vi "Cross Baseline.vi"(8 "error in (no error)":errorcluster, 9 "Scale Factor":sgl, 10 "Speed (ft/s)":dbl, 11 "Team Blue?":bool) -> (0 "error out":errorcluster)   [LabVIEW 2016]
uses:
  <vilib>/Rock Robotics/WPI/RobotDrive/WPI_RobotDriveMecanumDrive_Cartesian.vi
  Global 4.vi
  <vilib>/vision/NI_Vision_Development_Module.lvlib
panel:
  out "X Limit":i32
  out "Y Limit":i32
  out "BrightestY":i32
  out "BrightestX":i32
  out "Brightestness":u16
  in  "Control Brightness":u16
  in  "Target Brightness":u16
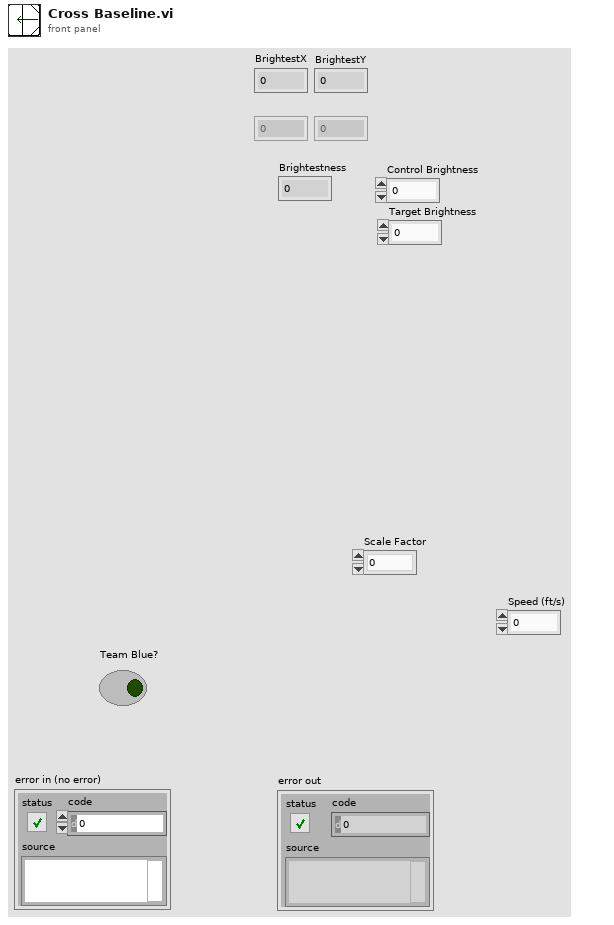
[diagram p1: front panel]
types:
  T1 = typedef "IMAQ Image.ctl" = refnum<image>
  T2 = typedef "WPI_RobotDriveDevRef.ctl" = cluster{"DevStatus":errorcluster, "Motors[]":T3[], "Square Inputs":bool, "Max Output":dbl}
  T3 = typedef "WPI_MotorControlDeviceRef.ctl" = cluster{"DeviceStatus":errorcluster, "Type":T4, "PWM":cluster{"PWM Channel":T5, "DeadBand":T6}, "CAN":cluster{"Device Number":u8, "SetOutput VI Ref":variant, "GetOutput VI Ref":variant, "Enable VI Ref":variant, "Disable VI Ref":variant, "Data":variant}, "Invert":bool}
  T4 = typedef "WPI_MotorControlType.ctl" = enum16{"PWM", "CAN"}
  T5 = typedef "FPGA_DIOPWMChannel.ctl" = enum8{"PWM 0", "PWM 1", "PWM 2", "PWM 3", "PWM 4", "PWM 5", "PWM 6", "PWM 7", "PWM 8", "PWM 9", "PWM MXP 0", "PWM MXP 1", "PWM MXP 2", "PWM MXP 3", "PWM MXP 4", "PWM MXP 5", "PWM MXP 6", "PWM MXP 7", "PWM MXP 8", "PWM MXP 9", "Invalid"}
  T6 = typedef "WPI_PWMDeadband.ctl" = cluster{"Name":string, "maxPositivePwm":i32, "minPositivePwm":i32, "centerPwm":i32, "maxNegativePwm":i32, "minNegativePwm":i32, "angularRange":u16}
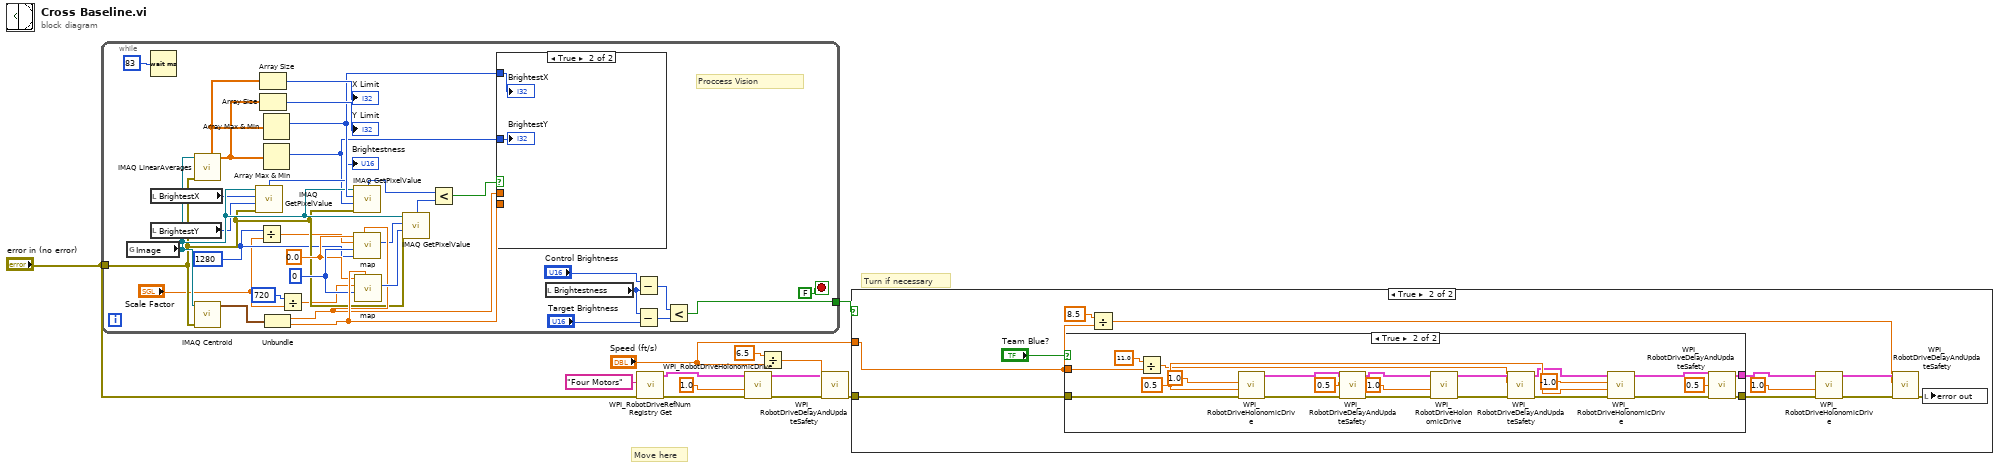
[diagram p0: block diagram]
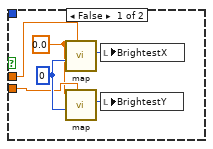
[diagram p2: hidden frame]
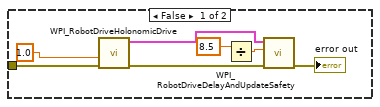
[diagram p3: hidden frame]
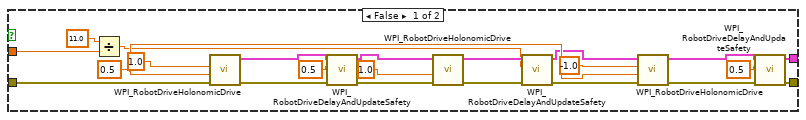
[diagram p4: hidden frame]
diagram:
  # "Turn if necessary"
  # "Move here"
  n1 = while {
    tunnel: "error in (no error)" -> [w19]
    tunnel: [w13] -> w12
    stop <- FALSE stop-if-true
    w17 = 1280
    w20 = sgl 0.0
    w21 = 0
    # "Proccess Vision"
    n2 = global read "Global 4.vi" "Image"() -> (w39:T1)
    n3 = Wait (ms)(milliseconds to wait=u32 83) -> ()  [unwired: 1 out]
    n4 = local read "BrightestX"() -> (w38:i32)
    n5 = local read "BrightestY"() -> (w37:i32)
    n6 = call "IMAQ LinearAverages"("error in (no error)"=w19, "Image Src"=w39) -> ("Y Axis Averages"=w42:sgl[], "X Axis Averages"=w43:sgl[])  [unwired: 5 in, 3 out]
    n7 = call "IMAQ Centroid"("error in (no error)"=w19, "Image"=w39) -> ("Centroid"=w44:cluster{"X Centroid":sgl, "Y Centroid":sgl})  [unwired: 2 in, 1 out]
    n8 = call "IMAQ GetPixelValue"("Image"=w39, "X Coordinate"=w38, "Y Coordinate"=w37, "error in (no error)"=w19) -> ("Pixel Value (U16)"=→"Brightestness":u16)  [unwired: 2 in, 4 out]
    n9 = Divide(x=w17, y="Scale Factor") -> (x/y=w18:sgl)
    n10 = Array Size(array=w43) -> (size(s)=→"X Limit":i32)
    n11 = Array Size(array=w42) -> (size(s)=→"Y Limit":i32)
    n12 = Array Max & Min(array=w43) -> (max index (indices)=w40:i32)  [unwired: 3 out]
    n13 = Array Max & Min(array=w42) -> (max index (indices)=w28:i32)  [unwired: 3 out]
    n14 = Unbundle(w44) -> ("X Centroid"=w23:sgl, "Y Centroid"=w25:sgl)
    n15 = Divide(x=720, y="Scale Factor") -> (x/y=w14:sgl)
    n16 = call "IMAQ GetPixelValue"("Image"=w39, "X Coordinate"=w40, "Y Coordinate"=w28, "error in (no error)"=w19) -> ("Pixel Value (U16)"=w33:u16)  [unwired: 2 in, 4 out]
    n17 = call "map.vi"("value"=w23, "newMax"=w17, "newMin"=w21, "oldMax"=w18, "oldMin"=w20) -> ("newValue"=w22:i32)  [unwired: 6 in]
    n18 = call "map.vi"("value"=w25, "newMin"=w21, "oldMax"=w14, "oldMin"=w20) -> ("newValue"=w24:i32)  [unwired: 7 in]
    n19 = call "IMAQ GetPixelValue"("Image"=w39, "X Coordinate"=w22, "Y Coordinate"=w24, "error in (no error)"=w19) -> ("Pixel Value (U16)"=w32:u16)  [unwired: 2 in, 4 out]
    n20 = Less?(x=w33, y=w32) -> (x < y?=w41:bool)
    n21 = case shown="True" w41 {
      tunnel: w40 -> [_ w54]
      tunnel: w23 -> [w52 _]
      tunnel: w25 -> [w49 _]
      tunnel: w28 -> [_ w53]
      frame False {
        w50 = 0
        w48 = sgl 0.0
        n22 = call "map.vi"("value"=w52, "newMin"=w50, "oldMin"=w48) -> ("newValue"=w51:i32)  [unwired: 8 in]
        n23 = call "map.vi"("value"=w49, "newMin"=w50, "oldMin"=w48) -> ("newValue"=w47:i32)  [unwired: 8 in]
        n24 = local write "BrightestX"(w51) -> ()
        n25 = local write "BrightestY"(w47) -> ()
      }
      frame True {
        "BrightestY" <- w53
        "BrightestX" <- w54
      }
    }
    n26 = local read "Brightestness"() -> (w36:u16)
    n27 = Subtract(x="Control Brightness", y=w36) -> (x-y=w29:u16)
    n28 = Subtract(x=w36, y="Target Brightness") -> (x-y=w30:u16)
    n29 = Less?(x=w29, y=w30) -> (x < y?=w13:bool)
  }
  n30 = call <vilib>:"WPI_RobotDriveRefNum Registry Get.vi"("error in (no error)"="error in (no error)", "refnum name"="Four Motors") -> ("error out"=w4:errorcluster, "RobotDriveDevRef"=w5:T2)  [unwired: 8 in]
  n31 = call-poly <vilib>:"WPI_RobotDriveHolonomicDrive.vi"("error in (no error)"=w4, "Y"=1.0, "RobotDriveDevRef"=w5) -> ("error out"=w9:errorcluster, "RobotDriveDevRef"=w8:T2)  [unwired: 6 in, 1 out]
  n32 = Divide(x=6.5, y="Speed (ft/s)") -> (x/y=w10:dbl)
  n33 = call <vilib>:"WPI_RobotDriveDelayAndUpdateSafety.vi"("error in (no error)"=w9, "Delay (s)"=w10, "RobotDriveDevRef"=w8) -> ("error out"=w2:errorcluster)  [unwired: 7 in, 1 out]
  n34 = case shown="True" w12 {
    tunnel: w2 -> [w57 w63]
    tunnel: "Speed (ft/s)" -> [_ w62]
    frame False {
      n35 = call-poly <vilib>:"WPI_RobotDriveHolonomicDrive.vi"("error in (no error)"=w57, "Y"=1.0) -> ("error out"=w60:errorcluster, "RobotDriveDevRef"=w59:T2)  [unwired: 7 in, 1 out]
      n36 = Divide(x=8.5) -> (x/y=w56:dbl)  [unwired: 1 in]
      n37 = call <vilib>:"WPI_RobotDriveDelayAndUpdateSafety.vi"("error in (no error)"=w60, "Delay (s)"=w56, "RobotDriveDevRef"=w59) -> ("error out"=→"error out":errorcluster)  [unwired: 7 in, 1 out]
    }
    frame True {
      n38 = case shown="True" "Team Blue?" {
        tunnel: [w79 w100] -> w72
        tunnel: [w78 w99] -> w71
        tunnel: w63 -> [w75 w97]
        tunnel: w62 -> [w73 w95]
        frame False {
          w84 = 0.5
          n39 = Divide(x=11.0, y=w73) -> (x/y=w76:dbl)
          n40 = call-poly <vilib>:"WPI_RobotDriveHolonomicDrive.vi"("error in (no error)"=w75, "Y"=w84, "X"=1.0) -> ("error out"=w90:errorcluster, "RobotDriveDevRef"=w91:T2)  [unwired: 6 in, 1 out]
          n41 = call <vilib>:"WPI_RobotDriveDelayAndUpdateSafety.vi"("error in (no error)"=w90, "Delay (s)"=0.5, "RobotDriveDevRef"=w91) -> ("error out"=w88:errorcluster, "RobotDriveDevRef 2"=w89:T2)  [unwired: 7 in]
          n42 = call-poly <vilib>:"WPI_RobotDriveHolonomicDrive.vi"("error in (no error)"=w88, "Y"=1.0, "RobotDriveDevRef"=w89) -> ("error out"=w85:errorcluster, "RobotDriveDevRef"=w86:T2)  [unwired: 6 in, 1 out]
          n43 = call <vilib>:"WPI_RobotDriveDelayAndUpdateSafety.vi"("error in (no error)"=w85, "Delay (s)"=w76, "RobotDriveDevRef"=w86) -> ("error out"=w82:errorcluster, "RobotDriveDevRef 2"=w83:T2)  [unwired: 7 in]
          n44 = call-poly <vilib>:"WPI_RobotDriveHolonomicDrive.vi"("error in (no error)"=w82, "Y"=w84, "X"=-1.0, "RobotDriveDevRef"=w83) -> ("error out"=w80:errorcluster, "RobotDriveDevRef"=w81:T2)  [unwired: 5 in, 1 out]
          n45 = call <vilib>:"WPI_RobotDriveDelayAndUpdateSafety.vi"("error in (no error)"=w80, "Delay (s)"=0.5, "RobotDriveDevRef"=w81) -> ("error out"=w78:errorcluster, "RobotDriveDevRef 2"=w79:T2)  [unwired: 7 in]
        }
        frame True {
          w106 = 0.5
          n46 = Divide(x=11.0, y=w95) -> (x/y=w98:dbl)
          n47 = call-poly <vilib>:"WPI_RobotDriveHolonomicDrive.vi"("error in (no error)"=w97, "Y"=w106, "X"=1.0) -> ("error out"=w112:errorcluster, "RobotDriveDevRef"=w113:T2)  [unwired: 6 in, 1 out]
          n48 = call <vilib>:"WPI_RobotDriveDelayAndUpdateSafety.vi"("error in (no error)"=w112, "Delay (s)"=0.5, "RobotDriveDevRef"=w113) -> ("error out"=w110:errorcluster, "RobotDriveDevRef 2"=w111:T2)  [unwired: 7 in]
          n49 = call-poly <vilib>:"WPI_RobotDriveHolonomicDrive.vi"("error in (no error)"=w110, "Y"=1.0, "RobotDriveDevRef"=w111) -> ("error out"=w107:errorcluster, "RobotDriveDevRef"=w108:T2)  [unwired: 6 in, 1 out]
          n50 = call <vilib>:"WPI_RobotDriveDelayAndUpdateSafety.vi"("error in (no error)"=w107, "Delay (s)"=w98, "RobotDriveDevRef"=w108) -> ("error out"=w104:errorcluster, "RobotDriveDevRef 2"=w105:T2)  [unwired: 7 in]
          n51 = call-poly <vilib>:"WPI_RobotDriveHolonomicDrive.vi"("error in (no error)"=w104, "Y"=w106, "X"=-1.0, "RobotDriveDevRef"=w105) -> ("error out"=w102:errorcluster, "RobotDriveDevRef"=w103:T2)  [unwired: 5 in, 1 out]
          n52 = call <vilib>:"WPI_RobotDriveDelayAndUpdateSafety.vi"("error in (no error)"=w102, "Delay (s)"=0.5, "RobotDriveDevRef"=w103) -> ("error out"=w99:errorcluster, "RobotDriveDevRef 2"=w100:T2)  [unwired: 7 in]
        }
      }
      n53 = Divide(x=8.5, y=w62) -> (x/y=w65:dbl)
      n54 = call-poly <vilib>:"WPI_RobotDriveHolonomicDrive.vi"("error in (no error)"=w71, "Y"=1.0, "RobotDriveDevRef"=w72) -> ("error out"=w67:errorcluster, "RobotDriveDevRef"=w68:T2)  [unwired: 6 in, 1 out]
      n55 = call <vilib>:"WPI_RobotDriveDelayAndUpdateSafety.vi"("error in (no error)"=w67, "Delay (s)"=w65, "RobotDriveDevRef"=w68) -> ("error out"=w66:errorcluster)  [unwired: 7 in, 1 out]
      n56 = local write "error out"(w66) -> ()
    }
  }
